vi "Read Scale Position.vi"(9 "RotaryColorScale in":refnum<class "RotaryColorScale.lvclass">) -> (3 "RotaryColorScale out":refnum<class "RotaryColorScale.lvclass">, 4 "Scale Position":T1)   [LabVIEW 2014, in "Raspberry Pi Compatible Compiler for LabVIEW.lvlib" / "RotaryColorScale.lvclass"]
uses:
  RotaryColorScale.lvclass
  <vilib>/Utility/miscctls.llb/LVScalePositionTypeDef.ctl
  RotaryColorScale.lvclass/RotaryColorScale.ctl
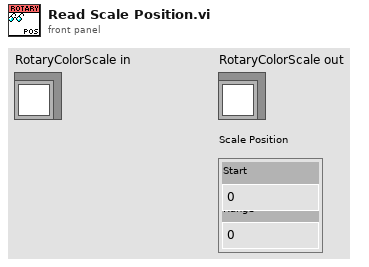
[diagram p1: front panel]
types:
  T1 = typedef "LVScalePositionTypeDef.ctl" = cluster{"Start":dbl, "Range":dbl}
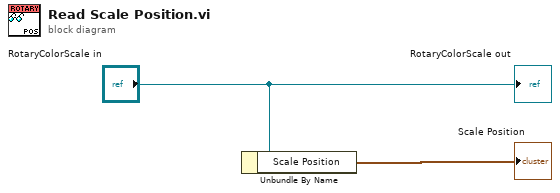
[diagram p0: block diagram]
diagram:
  n1 = Unbundle By Name("RotaryColorScale in") -> ("Scale Position"=→"Scale Position":T1)
  "RotaryColorScale out" <- "RotaryColorScale in"
